vi "AddBumpers.vi"(10 "Alliance":T1, 11 "Refnum in":T2) -> (3 "Refnum out":T2)   [LabVIEW 2019]
uses:
  <vilib>/vision/Image Controls.llb/IMAQ Image.ctl
  <vilib>/Rock Robotics/WPI/DriverStation/WPI_DriverStationAllianceInfo.ctl
  <vilib>/vision/NI_Vision_Development_Module.lvlib
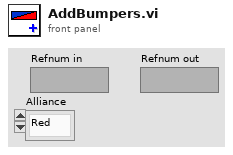
[diagram p1: front panel]
types:
  T1 = typedef "WPI_DriverStationAllianceInfo.ctl" = enum16{"Red", "Blue", "Invalid"}
  T2 = typedef "IMAQ Image.ctl" = refnum<image>
  T3 = typedef "Image Type" = u32
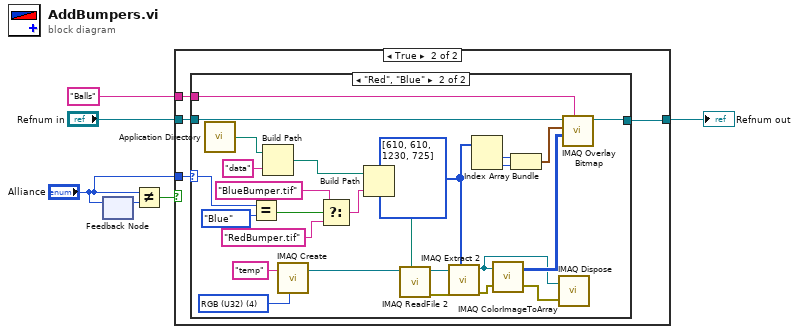
[diagram p0: block diagram]
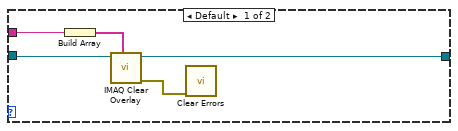
[diagram p3: hidden frame]
diagram:
  n1 = feedback-in #1("Alliance") -> ()
  n2 = feedback #1() -> (w5:T1)  [unwired: 1 in]
  n3 = Not Equal?(x="Alliance", y=w5) -> (x != y?=w6:bool)
  n4 = case shown="True" w6 {
    tunnel: [w7 w10] -> w4
    tunnel: "Refnum in" -> [w7 w11]
    tunnel: "Balls" -> [_ w9]
    tunnel: "Alliance" -> [_ w8]
    frame False {
    }
    frame True {
      n5 = case shown="\"Red\", \"Blue\"" w8 {
        selector: w8 -> [_ w22]
        tunnel: w11 -> [w16 w41]
        tunnel: [w15 w40] -> w10
        tunnel: w9 -> [w14 w42]
        frame Default {
          n6 = Build Array(w14) -> (w13:string[])
          n7 = call "IMAQ Clear Overlay"("Groups"=w13, "Image"=w16) -> ("error out"=w12:errorcluster, "Image Out"=w15:T2)  [unwired: 8 in]
          n8 = call <vilib>:"Clear Errors.vi"("error in (no error)"=w12) -> ()  [unwired: 5 in, 2 out]
        }
        frame "Red", "Blue" {
          w29 = i32[] [610, 610, 1230, 725] ("Optional Rectangle")
          w35 = T3 4 items=["Grayscale (U8)", "Grayscale (I16)", "Grayscale (SGL)", "Complex (CSG)", "RGB (U32)", "HSL (U32)", "RGB (U64)", "Grayscale (U16)"] ("Image Type")
          n9 = call <vilib>:"Application Directory.vi"() -> ("Application Directory"=w38:path)
          n10 = Equal?(x=w22, y=WPI_DriverStationAllianceInfo."Blue") -> (x = y?=w17:bool)
          n11 = Build Path(base path=w38, name or relative path="data") -> (appended path=w39:path)
          n12 = call "IMAQ Create"("Image Name"="temp", "Image Type"=w35) -> ("New Image"=w34:T2)  [unwired: 3 in, 1 out]
          n13 = Select(t="BlueBumper.tif" ("name or relative path"), s=w17, f="RedBumper.tif" ("name or relative path")) -> (s? t:f=w18:string)
          n14 = Build Path(base path=w39, name or relative path=w18) -> (appended path=w36:path)
          n15 = call "IMAQ ReadFile 2"("File Path"=w36, "Image"=w34) -> ("error out"=w33:errorcluster, "Image Out"=w32:T2)  [unwired: 5 in, 3 out]
          n16 = call "IMAQ Extract 2"("Optional Rectangle"=w29, "error in (no error)"=w33, "Image Src"=w32) -> ("error out"=w31:errorcluster, "Image Dst Out"=w24:T2)  [unwired: 7 in]
          n17 = Index Array(array=w29) -> (element #1=w27:i32, element #2=w28:i32)  [unwired: 2 in]
          n18 = call "IMAQ ColorImageToArray"("Image"=w24, "error in (no error)"=w31) -> ("Image Pixels (U32)"=w30:u32[][], "error out"=w25:errorcluster)  [unwired: 2 in, 1 out]
          n19 = Bundle(w27, w28) -> (w26:cluster{i32, i32})  [unwired: 1 in]
          n20 = call "IMAQ Dispose"("Image"=w24, "error in (no error)"=w25) -> ()  [unwired: 4 in, 1 out]
          n21 = call "IMAQ Overlay Bitmap"("Group"=w42, "Bitmap"=w30, "Top Left Point"=w26, "Image"=w41) -> ("Image Out"=w40:T2)  [unwired: 6 in, 1 out]
        }
      }
    }
  }
  "Refnum out" <- w4
